vi "Begin NI_XNET_CAN_Bus_Monitor_API StreamBus.vi"(6 "contextId":T1, 8 "error in":errorcluster, 9 "timeout (ms)":i32=-1, 10 "Request Data":T2, 11 "gRPC ID":T1) -> (0 "error out":errorcluster, 2 "Call Id Out":T1, 3 "gRPC ID out":T1)   [LabVIEW 2025, in "xnet_can_bus_monitor_api_client.lvlib"]
uses:
  xnet_can_bus_monitor_api_client.lvlib
  <vilib>/gRPC/LabVIEW gRPC Library/Shared/grpcId.ctl
  RPC Messages/ni_xnet_can_bm_api_StreamBusRequest.ctl
  59bd46bd-855a-43b3-a0b3-6a244c6a481b.vi
  <vilib>/gRPC/LabVIEW gRPC Library/Shared/TranslateGrpcError.vi
  <vilib>/gRPC/LabVIEW gRPC Library/Server API/Server/Get Server DLL Path.vi
  <vilib>/Utility/error.llb/Error Cluster From Error Code.vi
  <vilib>/gRPC/LabVIEW gRPC Library/grpc-lvsupport-release.lvlib
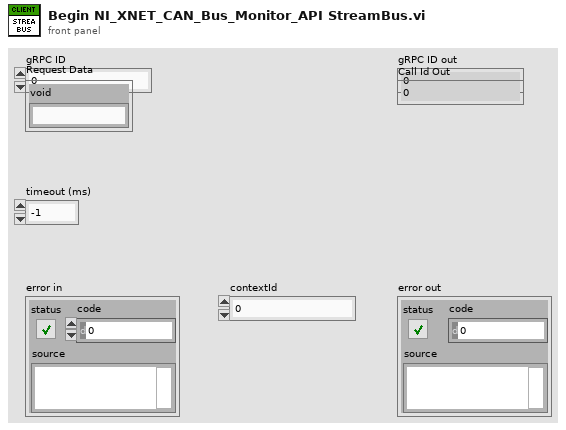
[diagram p1: front panel]
types:
  T1 = typedef "grpc-lvsupport-release.lvlib/grpcId.ctl" = u64
  T2 = typedef "xnet_can_bus_monitor_api_client.lvlib/ni_xnet_can_bm_api_StreamBusRequest.ctl" = cluster{"void":string}
  T3 = typedef "xnet_can_bus_monitor_api_client.lvlib/ni_xnet_can_bm_api_StreamBusRequest_Flat.ctl" = cluster{"void":string}
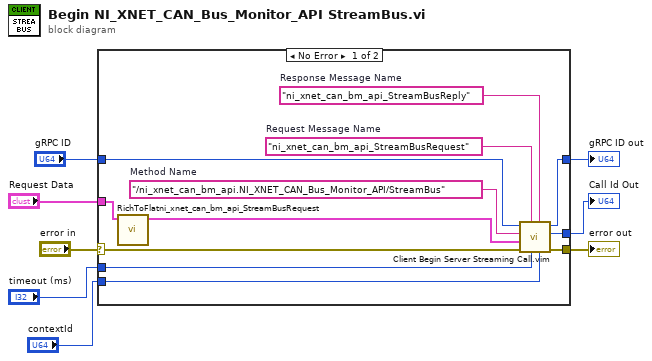
[diagram p0: block diagram]
diagram:
  n1 = case shown="No Error" "error in" {
    selector: "error in" -> [w17 w21]
    tunnel: [w16 w21] -> w7
    tunnel: "gRPC ID" -> [w15 w22]
    tunnel: [w14 w22] -> w5
    tunnel: [w13 _] -> w4
    tunnel: "Request Data" -> [w10 _]
    tunnel: "timeout (ms)" -> [w12 _]
    tunnel: "contextId" -> [w11 _]
    frame No Error {
      w18 = "ni_xnet_can_bm_api_StreamBusReply"  # Response Message Name
      w19 = "ni_xnet_can_bm_api_StreamBusRequest"  # Request Message Name
      w20 = "/ni_xnet_can_bm_api.NI_XNET_CAN_Bus_Monitor_API/StreamBus"  # Method Name
      n2 = call "RichToFlatni_xnet_can_bm_api_StreamBusRequest.vi"("InputCluster"=w10) -> ("OutputCluster"=w9:T3)  [unwired: 10 in]
      n3 = call "Client Begin Server Streaming Call.vim"("contextId"=w11, "Response Message Name"=w18, "timeout (ms)"=w12, "Request Message Name"=w19, "error in"=w17, "Request Data"=w9, "Method Name"=w20, "ClientID in"=w15) -> ("error out"=w16:errorcluster, "Call ID out"=w13:u64, "ClientID out"=w14:u64)  [unwired: 1 in]
    }
    frame Error {
    }
  }
  "error out" <- w7
  "gRPC ID out" <- w5
  "Call Id Out" <- w4
